vi "Profile Conversion.vi"() -> ()   [LabVIEW 2022 SP3]
panel:
  out "Numeric 2":i32
  out "Numeric":i32
  out "Timing Test":cluster{i32[], dbl[]}[](graph)
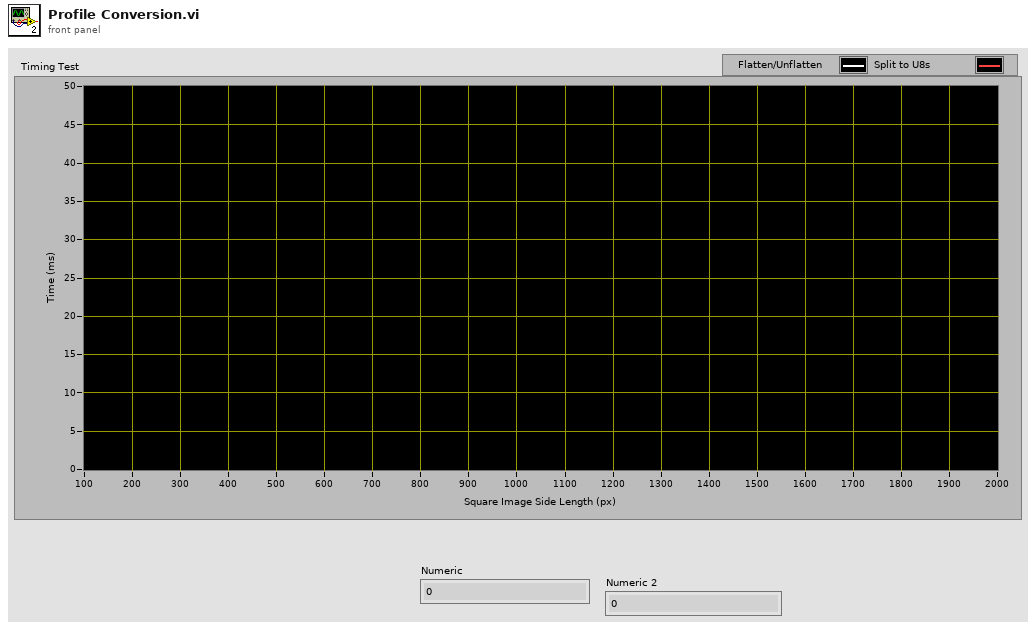
[diagram p1: front panel]
types:
  T1 = enum16{"big-endian, network order", "native, host order", "little-endian"}
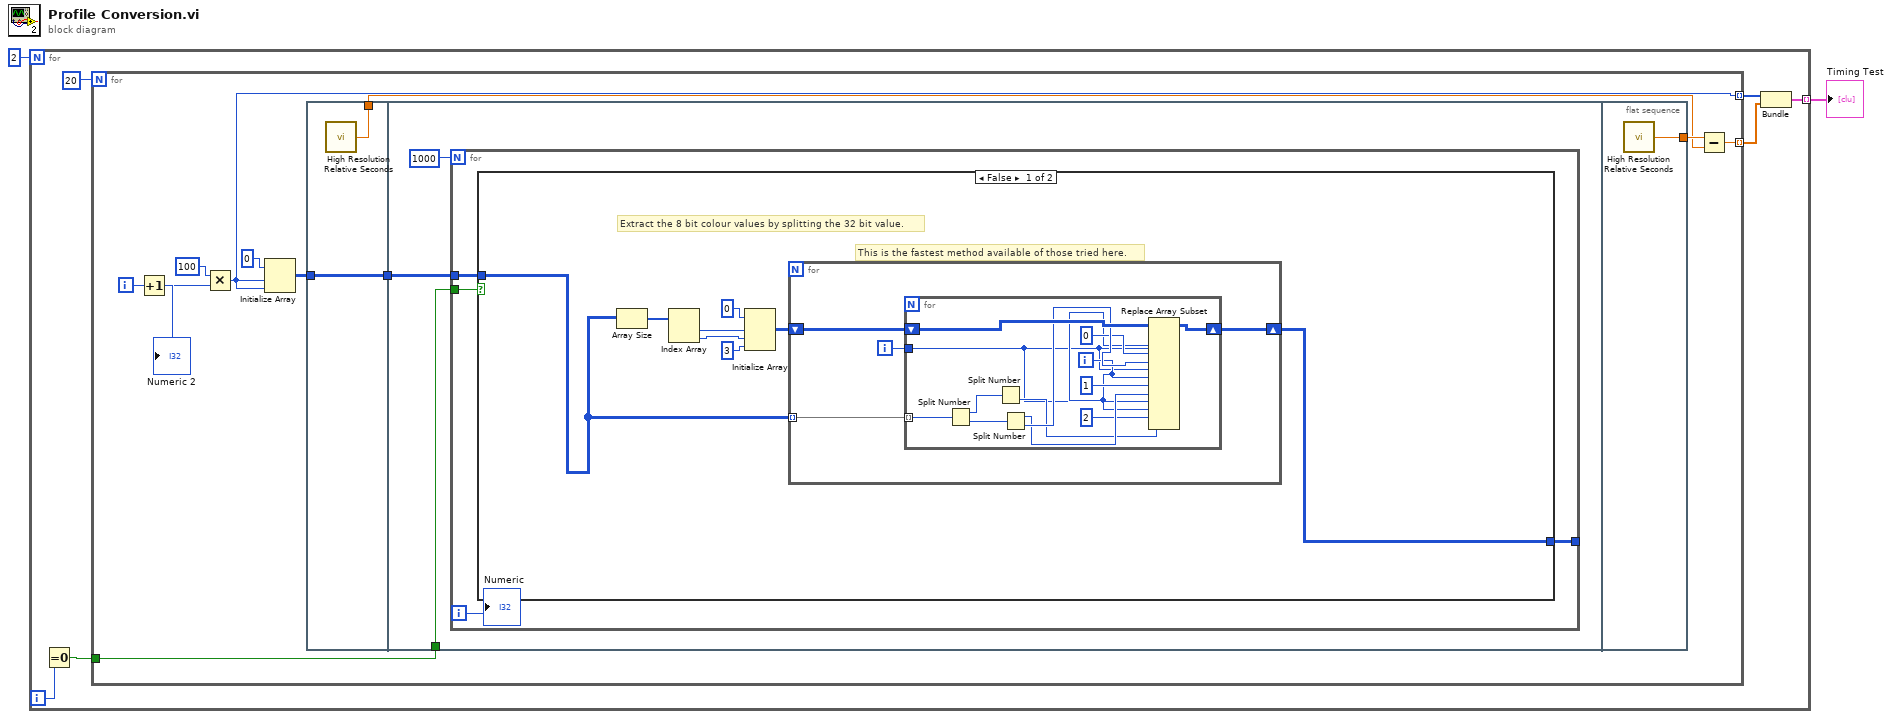
[diagram p0: block diagram]
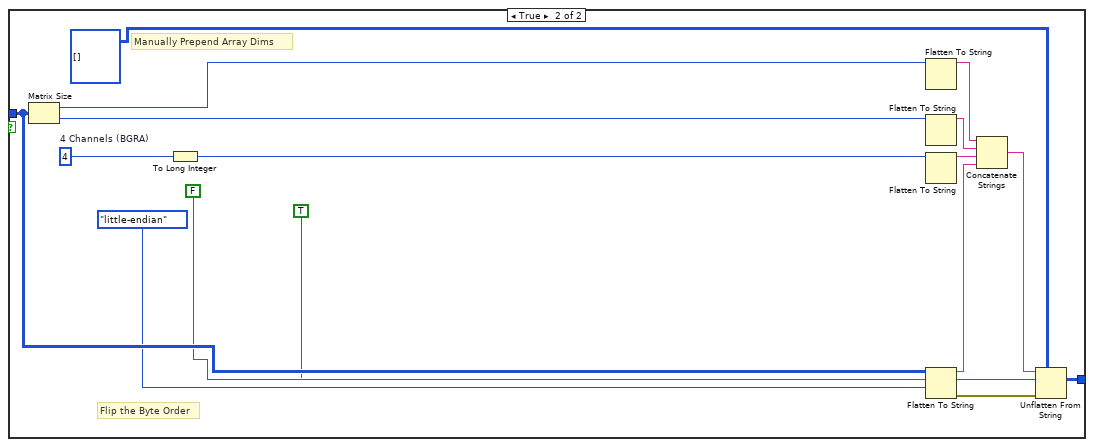
[diagram p2: hidden frame]
diagram:
  n1 = for {
    N: 2 -> [_]
    tunnel: [w5] -> w2 mode=indexing
    i -> [w4]
    n2 = Equal To 0?(x=w4) -> (x = 0?=w3:bool)
    n3 = for {
      N: 20 -> [_]
      tunnel: [w11] -> w6 mode=indexing
      tunnel: [w10] -> w7 mode=indexing
      tunnel: w3 -> [w9]
      i -> [w17]
      n4 = Increment(x=w17) -> (x+1=w15:i32)
      n5 = Multiply(x=100 ("dimension size"), y=w15) -> (x*y=w10:i32)
      n6 = Initialize Array(u32 0 ("element"), w10, w10) -> (w19:u32[][])
      n7 = flat-sequence {
        tunnel: w19 -> [w21]
        tunnel: [w21] -> w14
        tunnel: [w20] -> w12
        tunnel: w14 -> [w24]
        tunnel: w9 -> [w22]
        tunnel: [w70] -> w13
        frame #0 {
          n8 = call <vilib>:"High Resolution Relative Seconds.vi"() -> ("relative seconds"=w20:dbl)
        }
        frame #1 {
          n9 = for {
            N: 1000 -> [_]
            tunnel: w24 -> [w28]
            tunnel: [w27] -> _
            tunnel: w22 -> [w26]
            i -> [w25]
            n10 = case shown="False" w26 {
              tunnel: w28 -> [w36 w69]
              tunnel: [w29 w54] -> w27
              frame False {
                # "Extract the 8 bit colour values by splitting the 32 bit value."
                # "This is the fastest method available of those tried here."
                n11 = Array Size(array=w36) -> (size(s)=w35:i32[])
                n12 = Index Array(array=w35) -> (element #1=w34:i32, element #2=w33:i32)  [unwired: 2 in]
                n13 = Initialize Array(u8 0 ("dimension size"), w34, w33, 3 ("dimension size")) -> (w30:u8[][][])
                n14 = for {
                  tunnel: w36 -> [w40] mode=indexing
                  shift-right: [w38] -> w29
                  shift-left: w30 -> [w39]
                  i -> [w37]
                  n15 = for {
                    tunnel: w40 -> [w53] mode=indexing
                    shift-right: [w49] -> w38
                    shift-left: w39 -> [w50]
                    tunnel: w37 -> [w41]
                    i -> [w42]
                    n16 = Split Number(x=w53) -> (hi(x)=w52:u16, lo(x)=w51:u16)
                    n17 = Split Number(x=w52) -> (lo(x)=w46:u8)  [unwired: 1 out]
                    n18 = Split Number(x=w51) -> (hi(x)=w47:u8, lo(x)=w48:u8)
                    n19 = Replace Array Subset(array=w50, new element #1=w48, index (dim 0) #1=w41, index (dim 1) #1=w42, index (dim 2) #1=0 ("index (page)"), new element #2=w47, index (dim 0) #2=w41, index (dim 1) #2=w42, index (dim 2) #2=1 ("index (page)"), new element #3=w46, index (dim 0) #3=w41, index (dim 1) #3=w42, index (dim 2) #3=2 ("index (page)")) -> (w49:u8[][][])
                  }
                }
              }
              frame True {
                w63 = 4  # 4 Channels (BGRA)
                # "Flip the Byte Order"
                # "Manually Prepend Array Dims"
                n20 = Matrix Size(0:w69) -> (1:w64:i32, 2:w65:i32)
                n21 = To Long Integer(number=w63) -> (32bit integer=w62:i32)
                n22 = Flatten To String(anything=w64) -> (data string=w56:string)  [unwired: 3 in, 2 out]
                n23 = Flatten To String(anything=w65) -> (data string=w55:string)  [unwired: 3 in, 2 out]
                n24 = Flatten To String(anything=w62) -> (data string=w57:string)  [unwired: 3 in, 2 out]
                n25 = Flatten To String(anything=w69, prepend array or string size? (T)=FALSE, byte order (0:big-endian, network order)=T1."little-endian") -> (data string=w61:string, error out=w67:errorcluster)  [unwired: 1 in, 1 out]
                n26 = Concatenate Strings(w56, w55, w57, w61) -> (w60:string)
                n27 = Unflatten From String(type=u8[][][] [] ("Array"), binary string=w60, data includes array or string size? (T)=TRUE, error in (no error)=w67) -> (value=w54:u8[][][])  [unwired: 1 in, 2 out]
              }
            }
            "Numeric" <- w25
          }
        }
        frame #2 {
          n28 = call <vilib>:"High Resolution Relative Seconds.vi"() -> ("relative seconds"=w70:dbl)
        }
      }
      n29 = Subtract(x=w13, y=w12) -> (x-y=w11:dbl)
      "Numeric 2" <- w17
    }
    n30 = Bundle(w7, w6) -> (w5:cluster{i32[], dbl[]})  [unwired: 1 in]
  }
  "Timing Test" <- w2
